vi "LabView Project.vi"() -> ()   [LabVIEW 2021]
uses:
  <vilib>/sound2/lvsound2.llb/Sampling Mode.ctl
  <vilib>/sound2/lvsound2.llb/Sound Data Format.ctl
  Lab06/State Enum Type Def.ctl
  Analisys Type Def.ctl
  <vilib>/sound2/lvsound2.llb/Sound File Refnum.ctl
  <vilib>/Analysis/2dsp.llb/Power Spectrum (DBL).vi
  <vilib>/sound2/lvsound2.llb/Sound File Write (DBL).vi
  <vilib>/measure/maspectr.llb/FFT Power Spectrum and PSD for N Chan.vi
  <vilib>/sound2/lvsound2.llb/Sound File Write Open.vi
  <vilib>/sound2/lvsound2.llb/Sound Input Read (DBL).vi
  <vilib>/Analysis/NI_AALPro.lvlib
  <vilib>/measure/NI_MAPro.lvlib
panel:
  out "State":T1
  in  "?":enum32{"Recorded Signal", "Power Spectrum"}(tab)
  out "Sound Read Graph":waveform(dbl)[](graph)
  in  "Save Path":path
  out "Power Spectrum Chart":dbl[](graph)
  out "Power Spectrum Graph":cluster{"f0":dbl, "df":dbl, "magnitude":dbl[]}[](graph)
  in  "Exit Button":bool
  in  "Play Button":bool
  in  "Number of samples/ch":i32
  in  "Sound format":T2={"Sample Rate (S/s)"=22050.0, "Number of Channels"=2.0, "Bits Per Samples"=16.0} {"Bits Per Samples" min=0.0 max=64.0; "Number of Channels" min=1.0 max=2.0; "Sample Rate (S/s)" min=0.0}
  in  "Device":dbl
  in  "sample mode":T3 items=["Finite Samples", "Continuous Samples"]
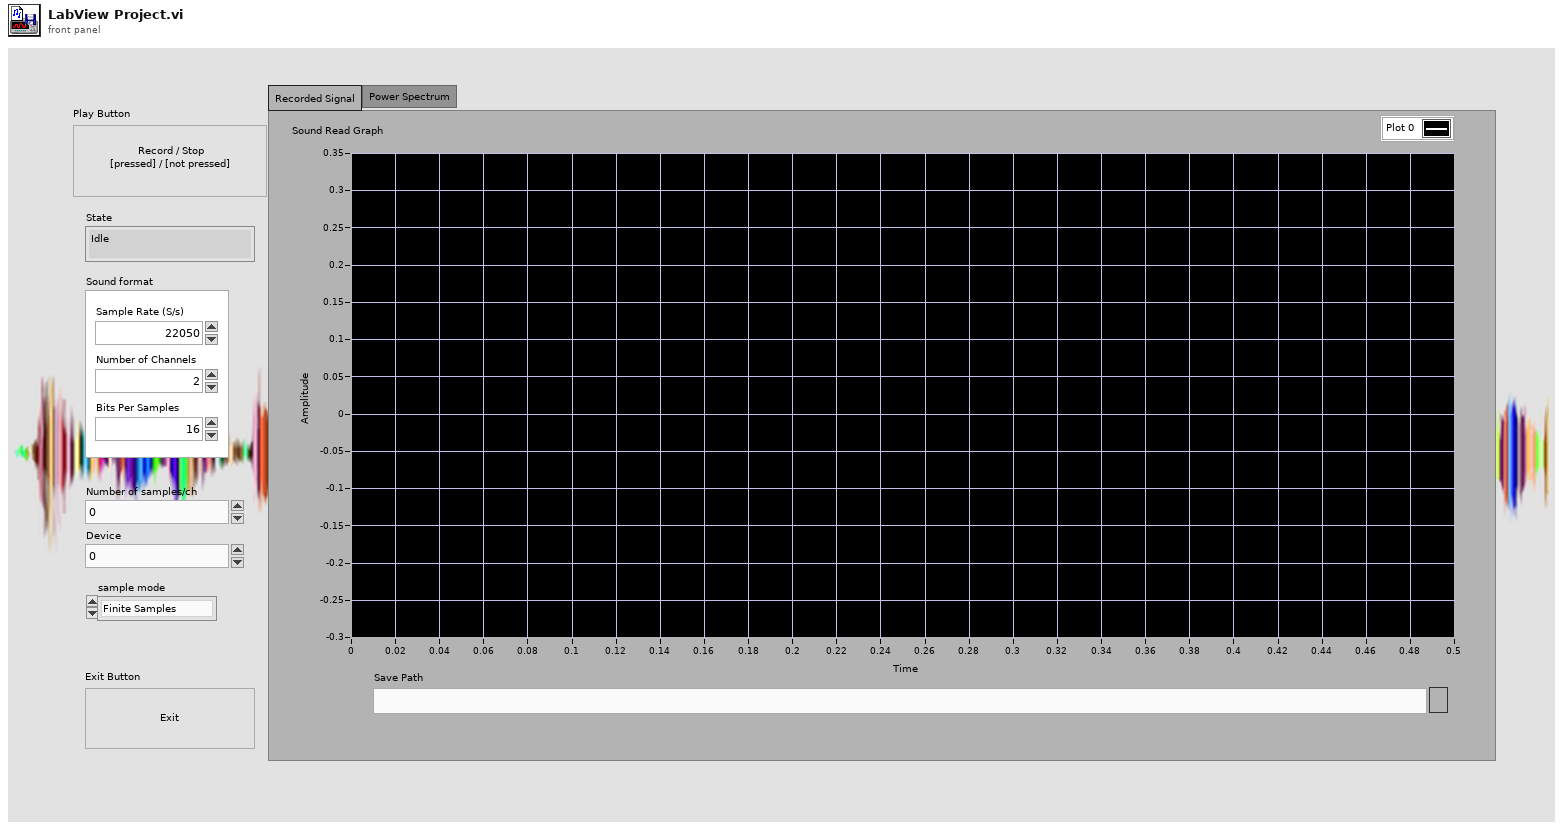
[diagram p1: front panel]
types:
  T1 = typedef "State Enum Type Def.ctl" = enum16{"Idle", "Init", "ACQ", "End"}
  T2 = typedef "Sound Data Format.ctl" = cluster{"Sample Rate (S/s)":dbl, "Number of Channels":dbl, "Bits Per Samples":dbl}
  T3 = typedef "Sampling Mode.ctl" = i32
  T4 = cluster{"Recorded Signal":waveform(dbl)[], "Power Spectrum":dbl[], "Power Spectrum / PSD":cluster{"f0":dbl, "df":dbl, "magnitude":dbl[]}[]}
  T5 = typedef "Analisys Type Def.ctl" = enum16{"Idle", "Create Save File", "Analysis State"}
  T6 = typedef "Sound File Refnum.ctl" = refnum<file>
  T7 = cluster{"Exit Button":bool, "Play Button":bool, "sound file refnum":T6}
  T8 = cluster{"sound format":T2, "number of samples/ch":i32, "Device":dbl, "sample mode":T3}
  T9 = typedef "Sound Input Task ID.ctl" = u32
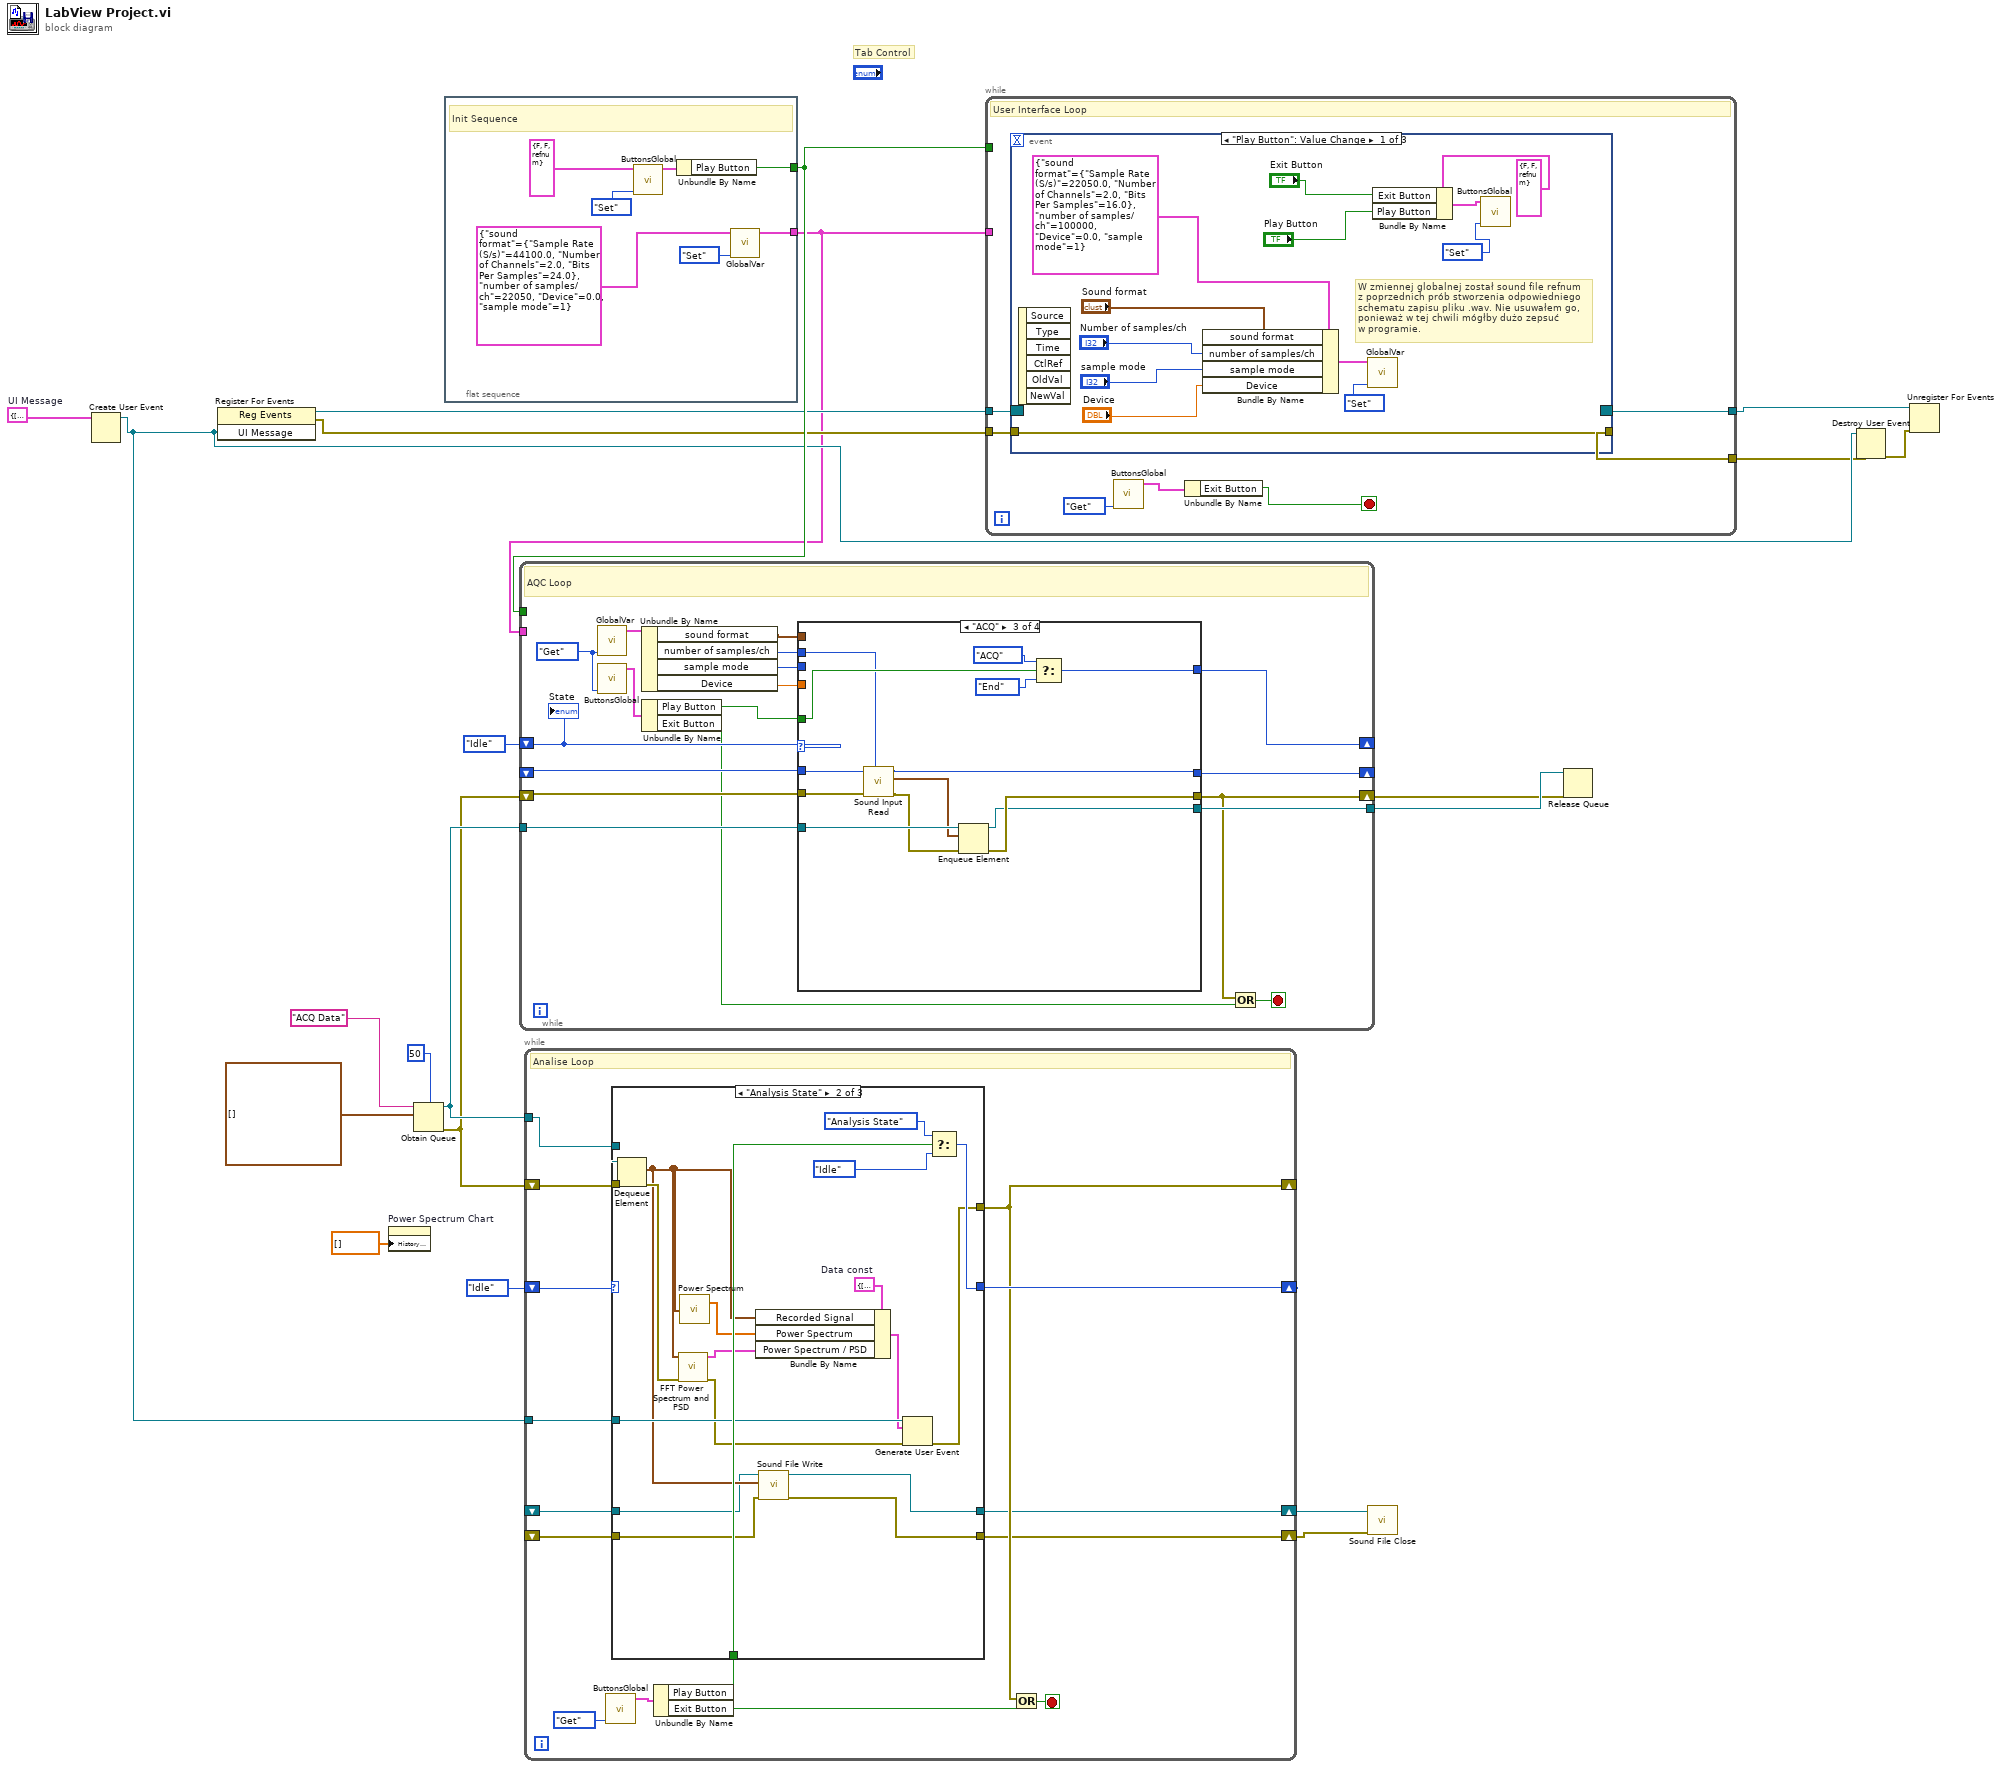
[diagram p0: block diagram]
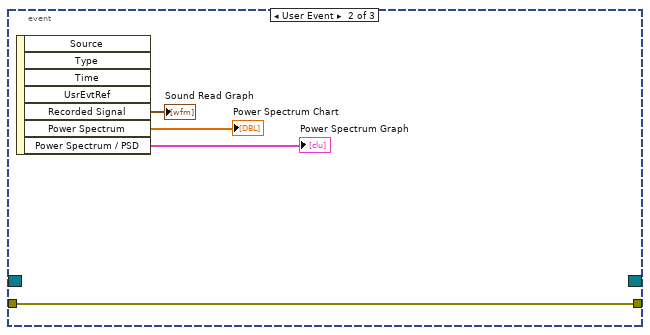
[diagram p2: hidden frame]
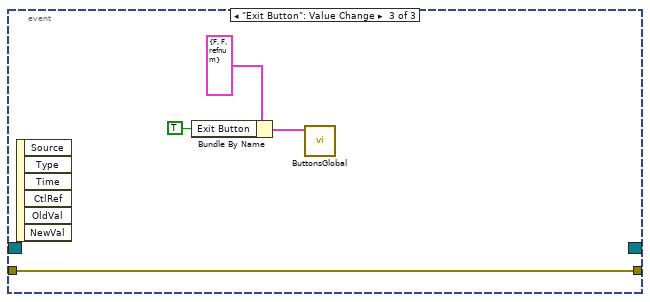
[diagram p3: hidden frame]
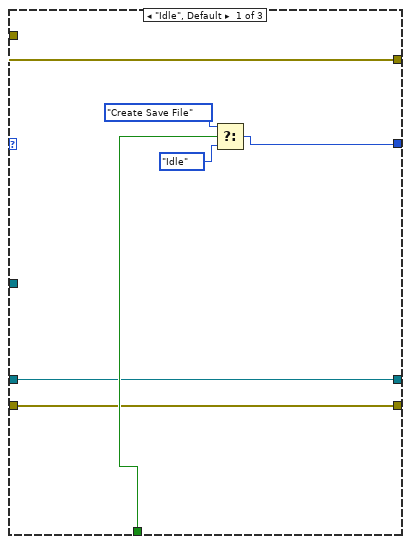
[diagram p4: hidden frame]
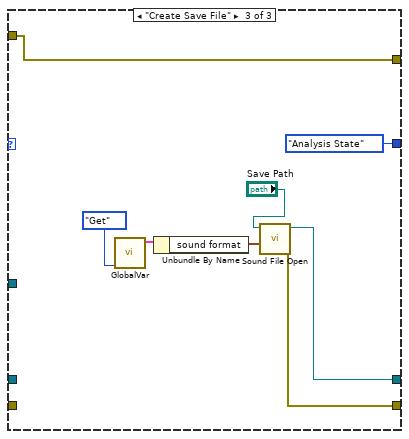
[diagram p5: hidden frame]
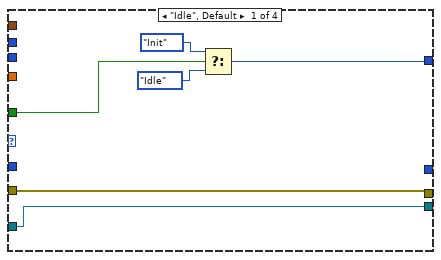
[diagram p6: hidden frame]
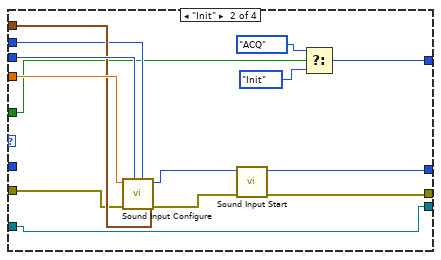
[diagram p7: hidden frame]
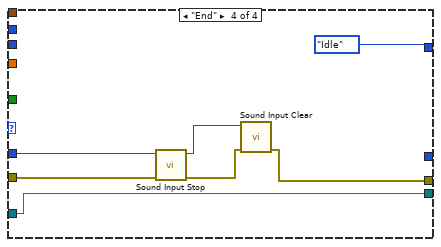
[diagram p8: hidden frame]
diagram:
  w10 = T4 {"Recorded Signal"=[], "Power Spectrum"=[], "Power Spectrum / PSD"=[]}  # UI Message
  # "Tab Control"
  n1 = Create User Event(user event datatype=w10) -> (user event=w7:refnum<user-event>)  [unwired: 1 in, 1 out]
  n2 = register-events(w7) -> (reference out=w11:refnum<event-registration>, error out=w9:errorcluster)  [unwired: 2 in]
  n3 = property on="Power Spectrum Chart" class="WFChart (strict)"("History Data"=dbl[] []) -> ()  [unwired: 2 in, 2 out]
  n4 = Obtain Queue(max queue size (-1, unlimited)=50, name (unnamed)="ACQ Data", element data type=waveform(dbl)[] [] ("data")) -> (queue out=w14:refnum<queue>, error out=w13:errorcluster)  [unwired: 2 in, 1 out]
  n5 = flat-sequence {
    tunnel: [w25] -> w16
    tunnel: [w24] -> w3
    frame #0 {
      # "Init Sequence"
      n6 = call "ButtonsGlobal.vi"("Action"=enum16{"Set", "Get"}."Set", "Input"=T7 {"Exit Button"=FALSE, "Play Button"=FALSE, "sound file refnum"=refnum}) -> ("Output"=w26:T7)  [unwired: 9 in]
      n7 = Unbundle By Name(w26) -> ("Play Button"=w25:bool)
      n8 = call "GlobalVar.vi"("Type Definition"=enum16{"Set", "Get"}."Set", "Param in"=T8 {"sound format"={"Sample Rate (S/s)"=44100.0, "Number of Channels"=2.0, "Bits Per Samples"=24.0}, "number of samples/ch"=22050, "Device"=0.0, "sample mode"=1}) -> ("Param out"=w24:T8)  [unwired: 9 in]
    }
  }
  n9 = while {
    shift-right: [w46] -> _
    shift-left: State_Enum_Type_Def."Idle" -> [w47]
    shift-right: [w45] -> _
    shift-left: _ -> [w44]
    shift-right: [w31] -> w4
    shift-left: w13 -> [w43]
    tunnel: [w34] -> _
    tunnel: w16 -> [w34]
    tunnel: [w33] -> w15
    tunnel: w14 -> [w32]
    tunnel: w3 -> [_]
    stop <- w29 stop-if-true
    w37 = enum16{"Set", "Get"}."Get" ("Type Definition")
    # "AQC Loop"
    n10 = call "GlobalVar.vi"("Type Definition"=w37) -> ("Param out"=w42:T8)  [unwired: 10 in]
    n11 = call "ButtonsGlobal.vi"("Action"=w37) -> ("Output"=w36:T7)  [unwired: 10 in]
    n12 = Unbundle By Name(w42) -> ("sound format"=w40:T2, "number of samples/ch"=w39:i32, "sample mode"=w38:T3, "Device"=w41:dbl)
    n13 = Unbundle By Name(w36) -> ("Play Button"=w35:bool, "Exit Button"=w30:bool)
    n14 = case shown="\"ACQ\"" w47 {
      tunnel: [w51 w65 w78 State_Enum_Type_Def."Idle"] -> w46
      tunnel: [w49 w56 w76 w82] -> w31
      tunnel: [_ w54 w72 _] -> w45
      tunnel: w44 -> [_ _ w73 w86]
      tunnel: w43 -> [w49 w57 w70 w87]
      tunnel: w41 -> [_ w62 _ _]
      tunnel: w38 -> [_ w61 _ _]
      tunnel: w40 -> [_ w60 _ _]
      tunnel: w39 -> [_ w59 w71 _]
      tunnel: w35 -> [w50 w58 w77 _]
      tunnel: [w48 w55 w75 w81] -> w33
      tunnel: w32 -> [w48 w55 w74 w81]
      frame "Idle", Default {
        n15 = Select(t=State_Enum_Type_Def."Init", s=w50, f=State_Enum_Type_Def."Idle") -> (s? t:f=w51:T1)
      }
      frame "Init" {
        n16 = call <vilib>:"Sound Input Configure.vi"("number of samples/ch"=w59, "sample mode"=w61, "error in (no error)"=w57, "sound format"=w60, "device ID"=w62) -> ("error out"=w66:errorcluster, "task ID"=w67:T9)  [unwired: 5 in]
        n17 = call <vilib>:"Sound Input Start.vi"("error in (no error)"=w66, "task ID"=w67) -> ("error out"=w56:errorcluster, "task ID out"=w54:T9)  [unwired: 8 in]
        n18 = Select(t=State_Enum_Type_Def."ACQ", s=w58, f=State_Enum_Type_Def."Init") -> (s? t:f=w65:T1)
      }
      frame "ACQ" {
        n19 = call-poly <vilib>:"Sound Input Read.vi"("number of samples/ch"=w71, "error in (no error)"=w70, "task ID"=w73) -> ("error out"=w69:errorcluster, "data"=w68:waveform(dbl)[], "task ID out"=w72:T9)  [unwired: 6 in]
        n20 = Enqueue Element(queue=w74, element=w68, error in (no error)=w69) -> (queue out=w75:refnum<queue>, error out=w76:errorcluster)  [unwired: 1 in, 1 out]
        n21 = Select(t=State_Enum_Type_Def."ACQ", s=w77, f=State_Enum_Type_Def."End") -> (s? t:f=w78:T1)
      }
      frame "End" {
        n22 = call <vilib>:"Sound Input Stop.vi"("error in (no error)"=w87, "task ID"=w86) -> ("error out"=w83:errorcluster, "task ID out"=w85:T9)  [unwired: 8 in]
        n23 = call <vilib>:"Sound Input Clear.vi"("error in (no error)"=w83, "task ID"=w85) -> ("error out"=w82:errorcluster)  [unwired: 9 in]
      }
    }
    n24 = Or(x=w31, y=w30) -> (x .or. y?=w29:bool)
    "State" <- w47
  }
  n25 = while {
    tunnel: w14 -> [w102]
    shift-right: [w96] -> _
    shift-left: Analisys_Type_Def."Idle" -> [w95]
    tunnel: w7 -> [w93]
    shift-right: [w92] -> _
    shift-left: w13 -> [w100]
    shift-right: [w90] -> w2
    shift-left: _ -> [w91]
    shift-right: [w89] -> w1
    shift-left: _ -> [w88]
    stop <- w101 stop-if-true
    # "Analise Loop"
    n26 = call "ButtonsGlobal.vi"("Action"=enum16{"Set", "Get"}."Get") -> ("Output"=w98:T7)  [unwired: 10 in]
    n27 = Unbundle By Name(w98) -> ("Play Button"=w94:bool, "Exit Button"=w97:bool)
    n28 = case shown="\"Analysis State\"" w95 {
      tunnel: w102 -> [_ w128 _]
      tunnel: [w106 w116 w129] -> w92
      tunnel: w100 -> [w106 w127 w129]
      tunnel: [w107 w124 Analisys_Type_Def."Analysis State"] -> w96
      tunnel: w94 -> [w105 w123 _]
      tunnel: w93 -> [_ w122 _]
      tunnel: [w104 w113 w130] -> w90
      tunnel: [w103 w112 w131] -> w89
      tunnel: w91 -> [w104 w111 _]
      tunnel: w88 -> [w103 w110 _]
      frame "Idle", Default {
        n29 = Select(t=Analisys_Type_Def."Create Save File", s=w105, f=Analisys_Type_Def."Idle") -> (s? t:f=w107:T5)
      }
      frame "Analysis State" {
        w121 = T4 {"Recorded Signal"=[], "Power Spectrum"=[], "Power Spectrum / PSD"=[]}  # Data const
        n30 = Dequeue Element(queue=w128, error in (no error)=w127) -> (element=w114:waveform(dbl)[], error out=w118:errorcluster)  [unwired: 1 in, 2 out]
        n31 = call-poly <vilib>:"FFT Power Spectrum and PSD.vi"("error in (no error)"=w118, "time signals"=w114) -> ("error out"=w117:errorcluster, "Power Spectrum / PSD"=w119:cluster{"f0":dbl, "df":dbl, "magnitude":dbl[]}[])  [unwired: 6 in, 2 out]
        n32 = call-poly <vilib>:"Power Spectrum.vi"("X"=w114) -> ("Power Spectrum"=w115:dbl[])  [unwired: 1 out]
        n33 = Bundle By Name(cluster=w121, "Recorded Signal"=w114, "Power Spectrum"=w115, "Power Spectrum / PSD"=w119) -> (w120:T4)
        n34 = call-poly <vilib>:"Sound File Write.vi"("error in (no error)"=w111, "data"=w114, "sound file refnum"=w110) -> ("error out"=w113:errorcluster, "sound file refnum out"=w112:T6)  [unwired: 7 in]
        n35 = Generate User Event(user event=w122, event data cluster=w120, error in=w117) -> (error out=w116:errorcluster)  [unwired: 1 in, 1 out]
        n36 = Select(t=Analisys_Type_Def."Analysis State", s=w123, f=Analisys_Type_Def."Idle") -> (s? t:f=w124:T5)
      }
      frame "Create Save File" {
        n37 = call "GlobalVar.vi"("Type Definition"=enum16{"Set", "Get"}."Get") -> ("Param out"=w135:T8)  [unwired: 10 in]
        n38 = Unbundle By Name(w135) -> ("sound format"=w136:T2)
        n39 = call-poly <vilib>:"Sound File Open.vi"("sound format"=w136, "path"="Save Path") -> ("error out"=w130:errorcluster, "sound file refnum"=w131:T6)  [unwired: 8 in]
      }
    }
    n40 = Or(x=w92, y=w97) -> (x .or. y?=w101:bool)
  }
  n41 = while {
    tunnel: w16 -> [_]
    tunnel: w11 -> [w140]
    tunnel: w9 -> [w139]
    tunnel: [w138] -> w8
    tunnel: [w137] -> w6
    tunnel: w3 -> [_]
    stop <- w141 stop-if-true
    # "User Interface Loop"
    n42 = event shown="[0] \"Play Button\": Value Change" {
      selector: w140 -> [_ _ _]
      dyn-events: [_ _ _] -> w138
      timeout: _ -> [_ _ _]
      tunnel: w139 -> [w148 w157 w163]
      tunnel: [w148 w157 w163] -> w137
      event "Play Button": Value Change {
        # "W zmiennej globalnej został sound file refnum\nz poprzednich prób stworzenia odpowiedniego\nschematu zapisu pliku .wav. Nie usuwałem go, \nponieważ w tej chwili mógłby dużo zepsuć\nw programie."
        n43 = event-data() -> ()  [unwired: 1 in, 6 out]
        n44 = Bundle By Name(cluster=T8 {"sound format"={"Sample Rate (S/s)"=22050.0, "Number of Channels"=2.0, "Bits Per Samples"=16.0}, "number of samples/ch"=100000, "Device"=0.0, "sample mode"=1} ("Param in"), "sound format"="Sound format", "number of samples/ch"="Number of samples/ch", "sample mode"="sample mode", "Device"="Device") -> (w146:T8)
        n45 = call "GlobalVar.vi"("Type Definition"=enum16{"Set", "Get"}."Set", "Param in"=w146) -> ()  [unwired: 9 in, 1 out]
        n46 = Bundle By Name(cluster=T7 {"Exit Button"=FALSE, "Play Button"=FALSE, "sound file refnum"=refnum} ("Input"), "Exit Button"="Exit Button", "Play Button"="Play Button") -> (w144:T7)
        n47 = call "ButtonsGlobal.vi"("Action"=enum16{"Set", "Get"}."Set", "Input"=w144) -> ()  [unwired: 9 in, 1 out]
      }
      event User Event {
        n48 = event-data() -> ("Recorded Signal"=→"Sound Read Graph":waveform(dbl)[], "Power Spectrum"=→"Power Spectrum Chart":dbl[], "Power Spectrum / PSD"=→"Power Spectrum Graph":cluster{"f0":dbl, "df":dbl, "magnitude":dbl[]}[])  [unwired: 1 in, 4 out]
      }
      event "Exit Button": Value Change {
        n49 = event-data() -> ()  [unwired: 1 in, 6 out]
        n50 = Bundle By Name(cluster=T7 {"Exit Button"=FALSE, "Play Button"=FALSE, "sound file refnum"=refnum} ("Input"), "Exit Button"=TRUE) -> (w161:T7)
        n51 = call "ButtonsGlobal.vi"("Input"=w161) -> ()  [unwired: 10 in, 1 out]
      }
    }
    n52 = call "ButtonsGlobal.vi"("Action"=enum16{"Set", "Get"}."Get") -> ("Output"=w143:T7)  [unwired: 10 in]
    n53 = Unbundle By Name(w143) -> ("Exit Button"=w141:bool)
  }
  n54 = call <vilib>:"Sound File Close.vi"("error in (no error)"=w2, "sound file refnum"=w1) -> ()  [unwired: 9 in, 1 out]
  n55 = Release Queue(queue=w15, error in (no error)=w4) -> ()  [unwired: 1 in, 3 out]
  n56 = Destroy User Event(user event=w7, error in=w6) -> (error out=w5:errorcluster)
  n57 = Unregister For Events(event registration refnum=w8, error in=w5) -> ()  [unwired: 1 out]
